vi "ManagerEventCreate.vi"(8 "error in (no error)":errorcluster, 11 "Manager In":u64 caption="Device In") -> (0 "error out":errorcluster, 2 "Event Registration Refnum":refnum<event-registration>, 3 "Manager Out":u64 caption="Device Out")   [LabVIEW 2012, in "Phidget Manager.lvlib"]
doc: "${AccelerationChange:CreateHeader}"
uses:
  <instrlib>/Phidgets/Phidget Manager/Phidget Manager.lvlib
  phidget22.dll
  <instrlib>/Phidgets/Phidget Common/Phidget Common.lvlib
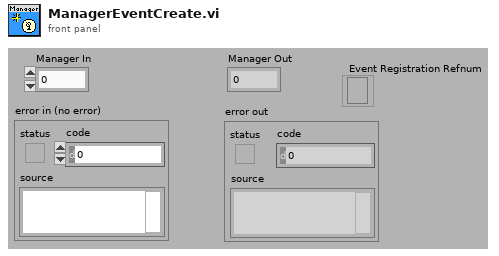
[diagram p1: front panel]
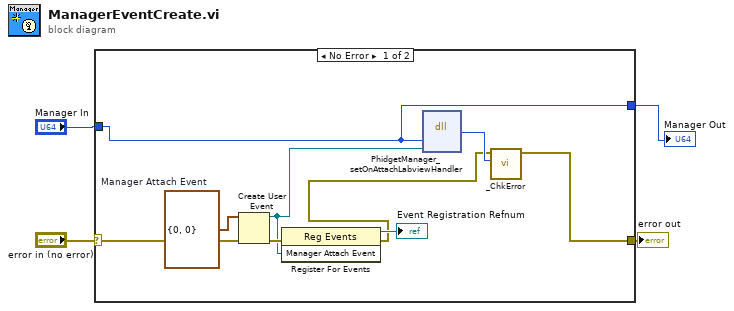
[diagram p0: block diagram]
diagram:
  n1 = case shown="No Error" "error in (no error)" {
    selector: "error in (no error)" -> [w13 w15]
    tunnel: [w5 w15] -> w3
    tunnel: "Manager In" -> [w6 w14]
    tunnel: [w6 w14] -> w1
    frame No Error {
      w11 = cluster{"manager":u64, "phid":u64} {"manager"=0, "phid"=0}  # Manager Attach Event
      n2 = Create User Event(user event datatype=w11, error in=w13) -> (user event=w7:refnum<user-event>, error out=w12:errorcluster)
      n3 = register-events(error in=w12, w7) -> (reference out=→"Event Registration Refnum":refnum<event-registration>, error out=w8:errorcluster)  [unwired: 1 in]
      n4 = dll-call lib="phidget22.*" fn="PhidgetManager_setOnAttachLabviewHandler"("phid"=w6, "AttachEvent"=w7) -> ("return type"=w9:i32)  [unwired: 5 in, 2 out]
      n5 = call <instrlib>:"_ChkError.vi"("Return Code"=w9, "error in (no error)"=w8) -> ("error out"=w5:errorcluster)  [unwired: 9 in]
    }
    frame Error {
    }
  }
  "error out" <- w3
  "Manager Out" <- w1
